vi "Assignment2_1.vi"() -> ()   [LabVIEW 2025]
doc: "This VI finds the Voltage failure point, below which the instrument does not work"
panel:
  out "Voltage_Failure_Point(V)":dbl
  in  "Voltage_Configurations":T1={"Minimum(V)"=3.0, "Maximum(V)"=5.0, "Resolution(V)"=0.01} {"Resolution(V)" min=0.01 max=0.01; "Maximum(V)" min=5.0 max=5.0; "Minimum(V)" min=3.0 max=3.0}
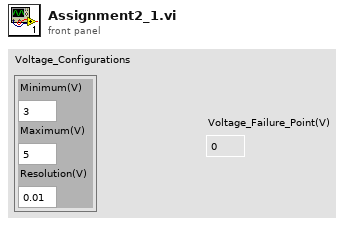
[diagram p1: front panel]
types:
  T1 = cluster{"Minimum(V)":dbl, "Maximum(V)":dbl, "Resolution(V)":dbl}
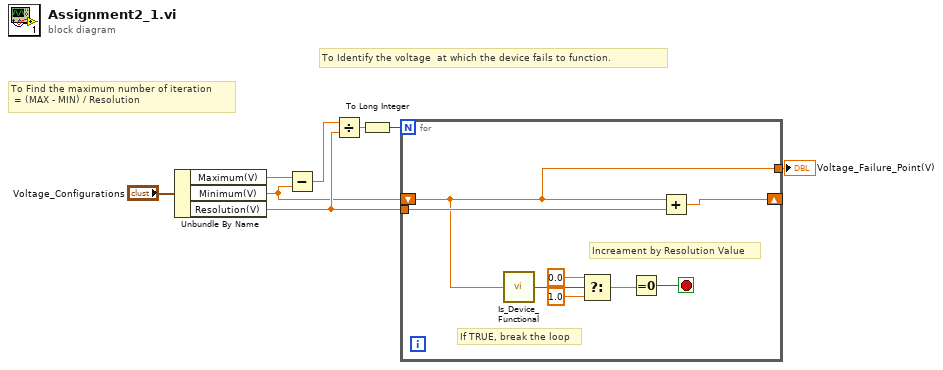
[diagram p0: block diagram]
diagram:
  # "To Find the maximum number of iteration\n = (MAX - MIN) / Resolution"
  # "To Identify the voltage  at which the device fails to function."
  n1 = Unbundle By Name("Voltage_Configurations") -> ("Maximum(V)"=w2:dbl, "Minimum(V)"=w1:dbl, "Resolution(V)"=w3:dbl)
  n2 = Subtract(x=w2, y=w1) -> (x-y=w7:dbl)
  n3 = Divide(x=w7, y=w3) -> (x/y=w6:dbl)
  n4 = To Long Integer(number=w6) -> (32bit integer=w5:i32)
  n5 = for {
    N: w5 -> [_]
    shift-right: [w15] -> _
    shift-left: w1 -> [w9]
    tunnel: w3 -> [w16]
    tunnel: [w9] -> w4
    stop <- w11 stop-if-true
    # "Increament by Resolution Value"
    # "If TRUE, break the loop"
    n6 = call "Is_Device_Functional.vi"("Operating_Voltage(V)"=w9) -> ("Device_Functional"=w14:bool)  [unwired: 14 in]
    n7 = Select(t=0.0, s=w14, f=1.0) -> (s? t:f=w12:dbl)
    n8 = Equal To 0?(x=w12) -> (x = 0?=w11:bool)
    n9 = Add(x=w9, y=w16) -> (x+y=w15:dbl)
  }
  "Voltage_Failure_Point(V)" <- w4
